vi "test_alignLeftValidation.vi"(11 "Test Case In":refnum<class "AlignmentTests.lvclass">) -> (0 "error out":errorcluster, 3 "Test Case Out":refnum<class "AlignmentTests.lvclass">)   [LabVIEW 2023, in "AlignmentTests.lvclass"]
uses:
  AlignmentTests.lvclass
  <vilib>/Astemes/LUnit/Test Case.lvclass/Test Case.ctl
  <vilib>/Astemes/LUnit/Core/LUnit Test Case/Private/Append Fail Result.vi
  <vilib>/Astemes/LUnit/Core/LUnit Test Case/Private/Append Pass Result.vi
  <vilib>/Astemes/LUnit/Core/LUnit Test Case/Private/Run In UI.vi
  <vilib>/Utility/error.llb/Clear Errors.vi
  AlignmentTests.lvclass/AlignmentTests.ctl
  <vilib>/Astemes/LUnit/Test Case.lvclass
panel:
  in  "Numeric 3":dbl
  in  "Numeric 2":dbl
  in  "Numeric":dbl
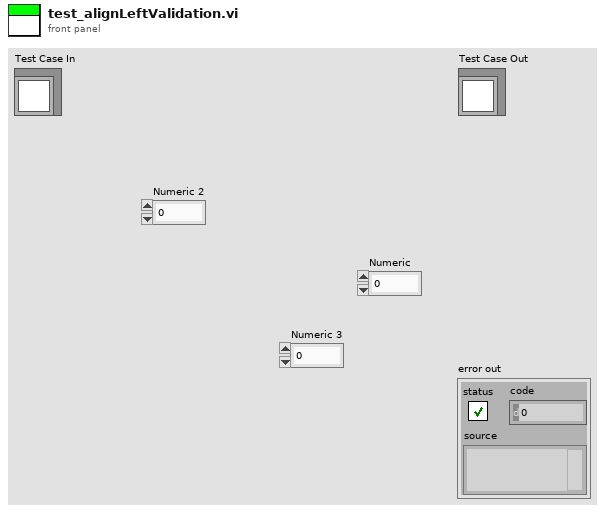
[diagram p1: front panel]
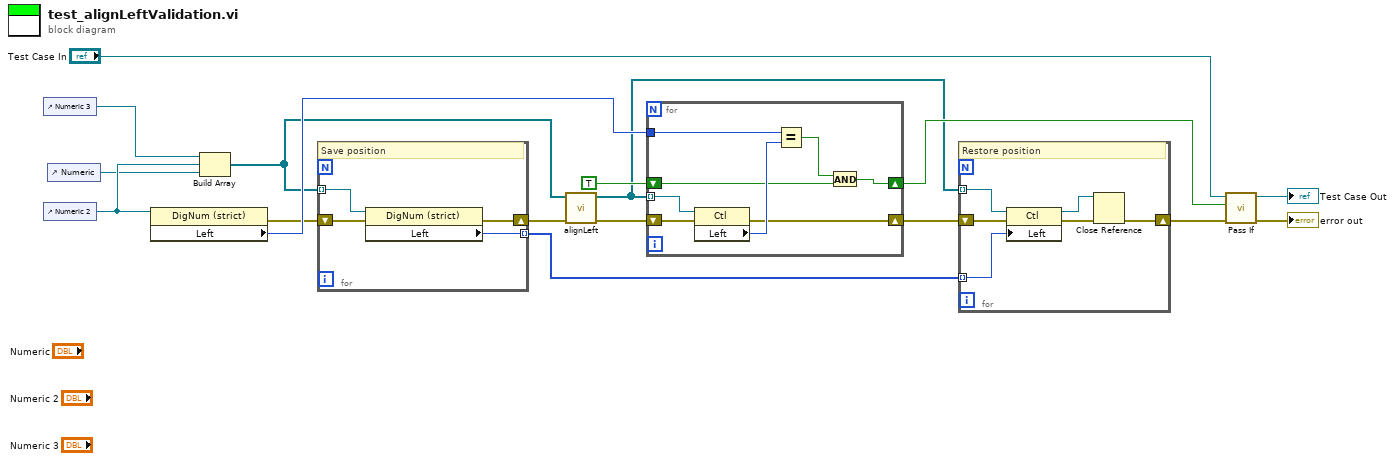
[diagram p0: block diagram]
diagram:
  n1 = control-ref of="Numeric 3"() -> (w14:refnum<vi>)
  n2 = control-ref of="Numeric 2"() -> (w13:refnum<vi>)
  n3 = control-ref of="Numeric"() -> (w12:refnum<vi>)
  n4 = property class="DigNum (strict)"(reference=w13) -> (error out=w7:errorcluster, "Left"=w11:i32)  [unwired: 1 in, 1 out]
  n5 = Build Array(w14, w13, w12) -> (w2:refnum<vi>[])
  n6 = for {
    tunnel: w2 -> [w21] mode=indexing
    shift-right: [w19] -> w6
    shift-left: w7 -> [w20]
    tunnel: [w18] -> w3 mode=indexing
    # "Save position"
    n7 = property class="DigNum (strict)"(reference=w21, error in=w20) -> (error out=w19:errorcluster, "Left"=w18:i32)  [unwired: 1 out]
  }
  n8 = call "alignLeft.vi"("error in (no error)"=w6, "refs"=w2) -> ("error out"=w8:errorcluster, "refs(dup)"=w1:refnum<vi>[])  [unwired: 8 in]
  n9 = for {
    tunnel: w1 -> [w29] mode=indexing
    tunnel: w11 -> [w27]
    shift-right: [w25] -> w9
    shift-left: TRUE -> [w24]
    shift-right: [w22] -> w4
    shift-left: w8 -> [w23]
    n10 = property class="Ctl"(reference=w29, error in=w23) -> (error out=w22:errorcluster, "Left"=w28:i32)  [unwired: 1 out]
    n11 = Equal?(x=w27, y=w28) -> (x = y?=w26:bool)
    n12 = And(x=w26, y=w24) -> (x .and. y?=w25:bool)
  }
  n13 = for {
    tunnel: w1 -> [w35] mode=indexing
    shift-right: [w31] -> w5
    shift-left: w4 -> [w34]
    tunnel: w3 -> [w32] mode=indexing
    # "Restore position"
    n14 = property class="Ctl"(reference=w35, error in=w34, "Left"=w32) -> (reference out=w30:refnum<vi>, error out=w33:errorcluster)
    n15 = Close Reference(reference=w30, error in (no error)=w33) -> (error out=w31:errorcluster)
  }
  n16 = call <vilib>:"Pass If.vi"("error in (no error)"=w5, "Pass?"=w9, "LUnit Test Case In"="Test Case In") -> ("error out"=→"error out":errorcluster, "LUnit Test Case Out"=→"Test Case Out":refnum<class "AlignmentTests.lvclass">)  [unwired: 7 in]
